vi "CS++Test.vi"() -> ()   [LabVIEW 2012]
uses:
  Core/Libraries/Base/CS++Base.lvlib
panel:
  out "found? 4":bool
  out "Array 2":variant[](array[variant])
  out "values":variant[](array[variant])
  out "Attributes":string[](array[string])
  out "Array":variant[](array[variant])
  out "found? 3":bool
  out "found? 2":bool
  out "found?":bool
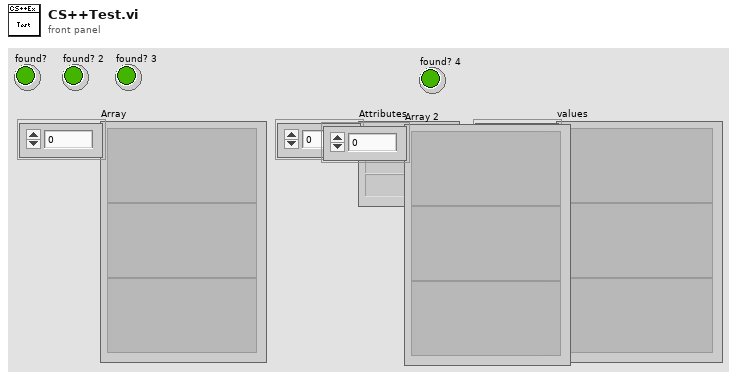
[diagram p1: front panel]
types:
  T1 = enum16{"add", "replace", "read", "remove", "reset", "get attibutes", ""}
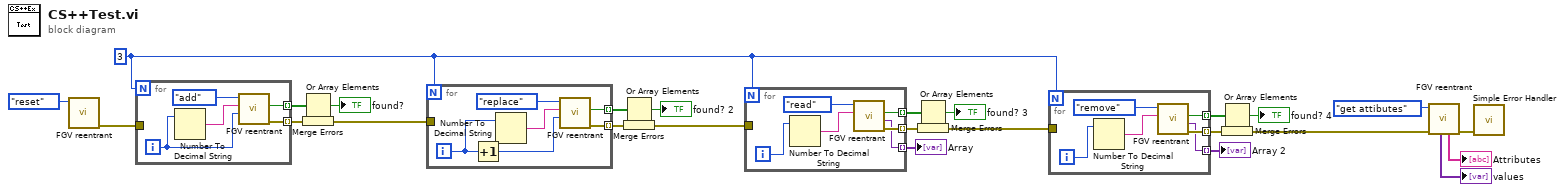
[diagram p0: block diagram]
diagram:
  w6 = 3
  n1 = call "FGV reentrant.vi"("Action (read)"=T1."reset") -> ("Error Out"=w2:errorcluster)  [unwired: 6 in, 4 out]
  n2 = for {
    N: w6 -> [_]
    tunnel: [w27] -> w25 mode=indexing
    tunnel: [w26] -> w24 mode=indexing
    tunnel: w2 -> [_]
    i -> [w29]
    n3 = Number To Decimal String(number=w29) -> (decimal integer string=w28:string)  [unwired: 1 in]
    n4 = call "FGV reentrant.vi"("Data"=w29, "Attribute Name"=w28, "Action (read)"=T1."add") -> ("Error Out"=w27:errorcluster, "found"=w26:bool)  [unwired: 4 in, 3 out]
  }
  n5 = Or Array Elements(Boolean array=w24) -> (logical OR=→"found?":bool)
  n6 = Merge Errors(w25) -> (w19:errorcluster)
  n7 = for {
    N: w6 -> [_]
    tunnel: [w34] -> w20 mode=indexing
    tunnel: [w33] -> w21 mode=indexing
    tunnel: w19 -> [_]
    i -> [w31]
    n8 = Increment(x=w31) -> (x+1=w32:i32)
    n9 = Number To Decimal String(number=w31) -> (decimal integer string=w35:string)  [unwired: 1 in]
    n10 = call "FGV reentrant.vi"("Data"=w32, "Attribute Name"=w35, "Action (read)"=T1."replace") -> ("Error Out"=w34:errorcluster, "found"=w33:bool)  [unwired: 4 in, 3 out]
  }
  n11 = Or Array Elements(Boolean array=w21) -> (logical OR=→"found? 2":bool)
  n12 = Merge Errors(w20) -> (w15:errorcluster)
  n13 = for {
    N: w6 -> [_]
    tunnel: [w40] -> w18 mode=indexing
    tunnel: [w39] -> w17 mode=indexing
    tunnel: w15 -> [_]
    tunnel: [w37] -> w14 mode=indexing
    i -> [w38]
    n14 = Number To Decimal String(number=w38) -> (decimal integer string=w41:string)  [unwired: 1 in]
    n15 = call "FGV reentrant.vi"("Attribute Name"=w41, "Action (read)"=T1."read") -> ("Error Out"=w40:errorcluster, "Data"=w37:variant, "found"=w39:bool)  [unwired: 5 in, 2 out]
  }
  "Array" <- w14
  n16 = Or Array Elements(Boolean array=w17) -> (logical OR=→"found? 3":bool)
  n17 = Merge Errors(w18) -> (w5:errorcluster)
  n18 = for {
    N: w6 -> [_]
    tunnel: [w46] -> w7 mode=indexing
    tunnel: [w45] -> w8 mode=indexing
    tunnel: [w43] -> w10 mode=indexing
    tunnel: w5 -> [_]
    i -> [w44]
    n19 = Number To Decimal String(number=w44) -> (decimal integer string=w47:string)  [unwired: 1 in]
    n20 = call "FGV reentrant.vi"("Attribute Name"=w47, "Action (read)"=T1."remove") -> ("Error Out"=w46:errorcluster, "Data"=w43:variant, "found"=w45:bool)  [unwired: 5 in, 2 out]
  }
  "Array 2" <- w10
  n21 = Or Array Elements(Boolean array=w8) -> (logical OR=→"found? 4":bool)
  n22 = Merge Errors(w7) -> (w4:errorcluster)
  n23 = call "FGV reentrant.vi"("Error In"=w4, "Action (read)"=T1."get attibutes") -> ("Error Out"=w3:errorcluster, "Attributes"=→"Attributes":string[], "values"=→"values":variant[])  [unwired: 5 in, 2 out]
  n24 = call <vilib>:"Simple Error Handler.vi"("error in (no error)"=w3) -> ()  [unwired: 4 in, 5 out]
